vi "HDPE State Machine Queue Driver.vi"(6 "Options":T2, 7 "Command":T1[](array[typedef]), 8 "error in (no error)":errorcluster, 11 "Queue Name":string="Main Event Loop Queue") -> (0 "error out":errorcluster, 1 "Queue Name":string, 2 "Timed Out?":bool, 3 "Queue Out":T1=enum.">Empty case", 4 "# Elements in Queue":i32)   [LabVIEW 2019]
uses:
  Controls/HDPE State Machine Cases.ctl
  Controls/HDPE State Machine Queue Driver Options.ctl
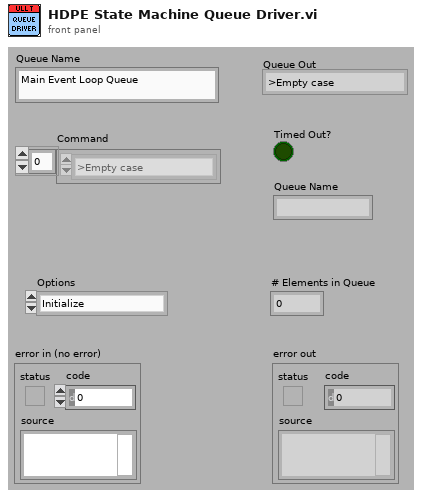
[diagram p1: front panel]
types:
  T1 = typedef "HDPE State Machine Cases.ctl" = enum16{">Poll", ">Init", ">Exit", ">Error", ">Empty case", ">Get Images", ">Control's State", ">Process Image", ">Open Index Image", ">Continuous"}
  T2 = typedef "HDPE State Machine Queue Driver Options.ctl" = enum16{"Initialize", "Get", "EnQ", "EnQ at Opp", "DeQ", "FlushQ", "Release", "Monitor Queue"}
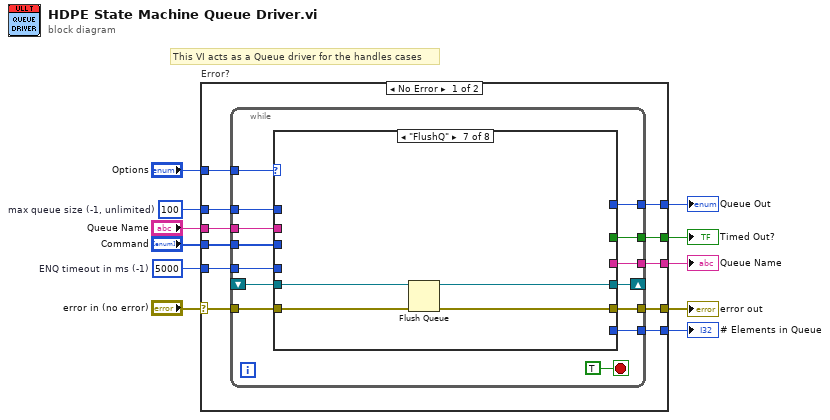
[diagram p0: block diagram]
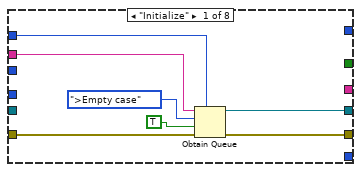
[diagram p2: hidden frame]
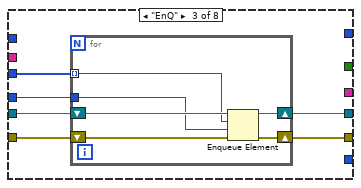
[diagram p4: hidden frame]
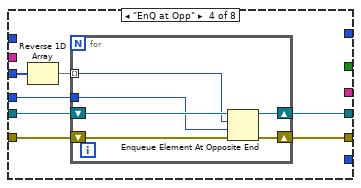
[diagram p5: hidden frame]
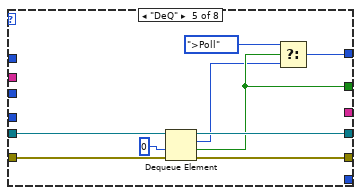
[diagram p6: hidden frame]
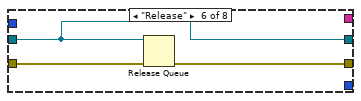
[diagram p7: hidden frame]
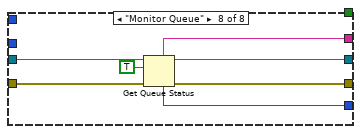
[diagram p8: hidden frame]
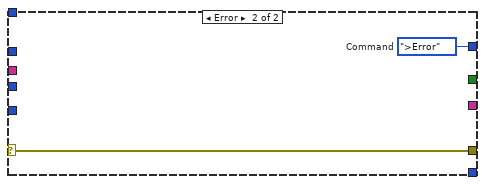
[diagram p9: hidden frame]
diagram:
  w2 = 5000  # ENQ timeout in ms (-1)
  w3 = 100  # max queue size (-1, unlimited)
  # "This VI acts as a Queue driver for the handles cases"
  n1 = case "Error?" shown="No Error" "error in (no error)" {
    selector: "error in (no error)" -> [w21 w95]
    tunnel: [w22 w95] -> w10
    tunnel: "Command" -> [w20 _]
    tunnel: "Options" -> [w19 _]
    tunnel: [w18 w94] -> w1
    tunnel: [w17 _] -> w7
    tunnel: "Queue Name" -> [w16 _]
    tunnel: [w15 _] -> w5
    tunnel: [w14 _] -> w4
    tunnel: w3 -> [w13 _]
    tunnel: w2 -> [w12 _]
    frame No Error {
      n2 = while {
        tunnel: [w33] -> w22
        tunnel: w21 -> [w31]
        tunnel: w20 -> [w35]
        shift-right: [w34] -> _
        shift-left: _ -> [w32]
        tunnel: w19 -> [w30]
        tunnel: [w29] -> w18
        tunnel: [w28] -> w17
        tunnel: w16 -> [w27]
        tunnel: [w26] -> w15
        tunnel: [w25] -> w14
        tunnel: w13 -> [w24]
        tunnel: w12 -> [w23]
        stop <- TRUE stop-if-true
        n3 = case shown="\"FlushQ\"" w30 {
          tunnel: w32 -> [_ w45 w51 w64 w78 w80 w84 w91]
          tunnel: w35 -> [_ _ w50 w63 _ _ _ _]
          tunnel: w31 -> [w37 w44 w49 w62 w77 w82 w86 w93]
          tunnel: [w41 w45 w48 w61 w75 w80 w83 w90] -> w34
          tunnel: [w40 w44 w47 w60 w76 w81 w85 w92] -> w33
          tunnel: [_ _ _ _ w71 _ _ _] -> w29
          tunnel: [_ _ _ _ w74 _ _ _] -> w28
          tunnel: w27 -> [w42 _ _ _ _ _ _ _]
          tunnel: [_ _ _ _ _ _ _ w88] -> w26
          tunnel: [_ _ _ _ _ _ _ w87] -> w25
          tunnel: w24 -> [w39 _ _ _ _ _ _ _]
          tunnel: w23 -> [_ _ w46 w59 _ _ _ _]
          frame "Initialize" {
            n4 = Obtain Queue(max queue size (-1, unlimited)=w39, name (unnamed)=w42, element data type=HDPE_State_Machine_Cases.">Empty case" ("Command"), create if not found? (T)=TRUE, error in (no error)=w37) -> (queue out=w41:refnum<queue>, error out=w40:errorcluster)  [unwired: 1 out]
          }
          frame "Get" {
          }
          frame "EnQ" {
            n5 = for {
              tunnel: w50 -> [w52] mode=indexing
              shift-right: [w56] -> w48
              shift-left: w51 -> [w54]
              shift-right: [w57] -> w47
              shift-left: w49 -> [w55]
              tunnel: w46 -> [w53]
              n6 = Enqueue Element(queue=w54, element=w52, timeout in ms (-1)=w53, error in (no error)=w55) -> (queue out=w56:refnum<queue>, error out=w57:errorcluster)  [unwired: 1 out]
            }
          }
          frame "EnQ at Opp" {
            n7 = Reverse 1D Array(array=w63) -> (reversed array=w58:T1[])
            n8 = for {
              tunnel: w58 -> [w65] mode=indexing
              shift-right: [w69] -> w61
              shift-left: w64 -> [w67]
              shift-right: [w70] -> w60
              shift-left: w62 -> [w68]
              tunnel: w59 -> [w66]
              n9 = Enqueue Element At Opposite End(queue=w67, element=w65, timeout in ms (-1)=w66, error in (no error)=w68) -> (queue out=w69:refnum<queue>, error out=w70:errorcluster)  [unwired: 1 out]
            }
          }
          frame "DeQ" {
            n10 = Dequeue Element(queue=w78, timeout in ms (-1)=0 ("ms timeout (-1)"), error in (no error)=w77) -> (queue out=w75:refnum<queue>, element=w72:T1, timed out?=w74:bool, error out=w76:errorcluster)
            n11 = Select(t=HDPE_State_Machine_Cases.">Poll", s=w74, f=w72) -> (s? t:f=w71:T1)
          }
          frame "Release" {
            n12 = Release Queue(queue=w80, error in (no error)=w82) -> (error out=w81:errorcluster)  [unwired: 1 in, 2 out]
          }
          frame "FlushQ" {
            n13 = Flush Queue(queue=w84, error in (no error)=w86) -> (queue out=w83:refnum<queue>, error out=w85:errorcluster)  [unwired: 1 out]
          }
          frame "Monitor Queue" {
            n14 = Get Queue Status(queue=w91, return elements? (F)=TRUE, error in (no error)=w93) -> (queue out=w90:refnum<queue>, queue name=w87:string, error out=w92:errorcluster, # elements in queue=w88:i32)  [unwired: 4 out]
          }
        }
      }
    }
    frame Error {
      w94 = HDPE_State_Machine_Cases.">Error"  # Command
    }
  }
  "error out" <- w10
  "Timed Out?" <- w7
  "# Elements in Queue" <- w5
  "Queue Name" <- w4
  "Queue Out" <- w1
